vi "PCO_GetROI.vi"(8 "error in (no error)":errorcluster {"code" format="%x"}, 11 "ph":u64) -> (0 "error out":errorcluster {"code" format="%x"}, 1 "wRoiX0":u16, 2 "ErrorMessage":i32 format="%x", 3 "ph out":u64, 4 "wRoiX1":u16, 5 "wRoiY0":u16, 7 "wRoiY1":u16)   [LabVIEW 2020, in "SDK.lvlib" / "ImageSensor.lvlib"]
doc: "<b>Description:</b>\nThis function returns the current ROI (region of interest) setting in pixels, see figure. If Soft ROI is enabled (see PCO_EnableSoftROI) the current setting of the Soft ROI are returned otherwise the ROI registers in the camera are readout.\nThe returned ROI is always equal to or smaller than the active image area, which is defined by the settings of format and binning (see chapter IMAGE AREA SELECTION (ROI) ).\n\n<b>Supported camera type:</b>\nAll cameras\n\n<b>Descriptor dependency:</b>\nwRoiHorStepsDESC, wRoiVertStepsDESC"
uses:
  ImageSensor.lvlib
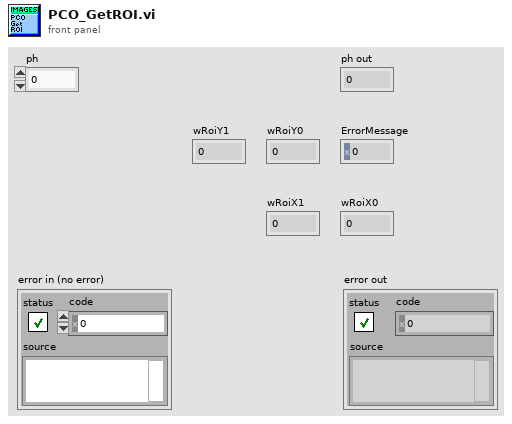
[diagram p1: front panel]
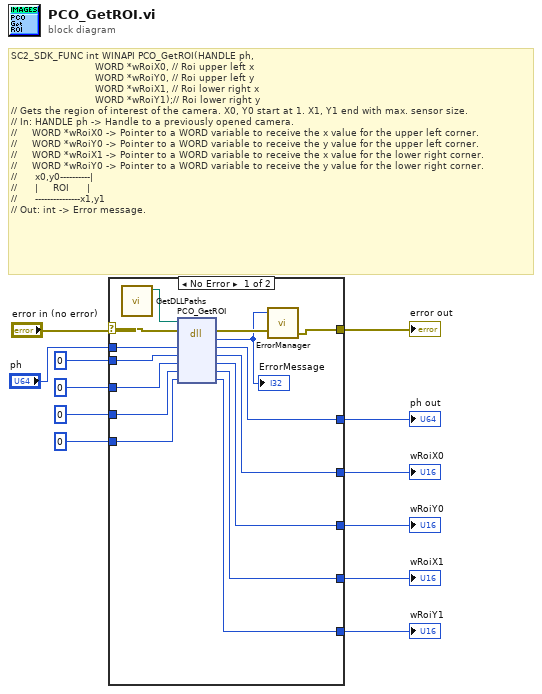
[diagram p0: block diagram]
diagram:
  # "SC2_SDK_FUNC int WINAPI PCO_GetROI(HANDLE ph,\n                            WORD *wRoiX0, // Roi upper left x\n                            WORD *wRoiY0, // Roi upper left y\n                            WORD *wRoiX1, // Roi lower right x\n                            WORD *wRoiY1);// Roi lower right y\n// Gets the region of interest of the camera. X0, Y0 start at 1. X1, Y1 end with max. sensor size.\n// In: HANDLE ph -> Handle to a previously opened camera.\n//     WORD *wRoiX0 -> Pointer to a WORD variable to receive the x value for the upper left corner.\n//     WORD *wRoiY0 -> Pointer to a WORD variable to receive the y value for the upper left corner.\n//     WORD *wRoiX1 -> Pointer to a WORD variable to receive the x value for the lower right corner.\n//     WORD *wRoiY0 -> Pointer to a WORD variable to receive the y value for the lower right corner.\n//      x0,y0----------|\n//      |     ROI      |\n//      ---------------x1,y1\n// Out: int -> Error message."
  n1 = case shown="No Error" "error in (no error)" {
    selector: "error in (no error)" -> [w15 w33]
    tunnel: "ph" -> [w27 w32]
    tunnel: [w26 w32] -> w11
    tunnel: u16 0 ("wRoiX0") -> [w25 w31]
    tunnel: [w24 w31] -> w9
    tunnel: u16 0 ("wRoiY0") -> [w23 w30]
    tunnel: [w22 w30] -> w7
    tunnel: u16 0 ("wRoiX1") -> [w21 w29]
    tunnel: [w20 w29] -> w5
    tunnel: u16 0 ("wRoiY1") -> [w19 w28]
    tunnel: [w18 w28] -> w3
    tunnel: [w16 w33] -> w2
    frame No Error {
      n2 = call "GetDLLPaths.vi"() -> ("SC2_Cam_Path"=w13:path)  [unwired: 9 in, 2 out]
      n3 = dll-call lib="?" fn="PCO_GetROI"(path in=w13, error in=w15, "ph"=w27, "wRoiX0"=w25, "wRoiY0"=w23, "wRoiX1"=w21, "wRoiY1"=w19) -> (error out=w17:errorcluster, "return type"=w14:i32, "ph"=w26:u64, "wRoiX0"=w24:u16, "wRoiY0"=w22:u16, "wRoiX1"=w20:u16, "wRoiY1"=w18:u16)  [unwired: 1 in, 1 out]
      "ErrorMessage" <- w14
      n4 = call "ErrorManager.vi"("error in (no error)"=w17, "error code"=w14) -> ("error out"=w16:errorcluster)  [unwired: 3 in]
    }
    frame Error {
    }
  }
  "ph out" <- w11
  "wRoiX0" <- w9
  "wRoiY0" <- w7
  "wRoiX1" <- w5
  "wRoiY1" <- w3
  "error out" <- w2
